vi "Write Handle Drag Starting Msg.vi"(6 "Handle Drag Starting Msg":refnum<class "Handle Drag Starting Msg.lvclass">, 11 "File Explorer Event Filter in":refnum<class "File Explorer Event Filter.lvclass">) -> (3 "File Explorer Event Filter out":refnum<class "File Explorer Event Filter.lvclass">)   [LabVIEW 2020, in "File Explorer.lvlib" / "File Explorer Event Filter.lvclass"]
uses:
  <vilib>/gpm_packages/@cs/file-explorer-extension/Source/File Explorer/File Explorer Event Filter/File Explorer Event Filter.lvclass
  <vilib>/gpm_packages/@cs/file-explorer-extension/Source/File Explorer/File Explorer Messages/Handle Drag Starting Msg/Handle Drag Starting Msg.lvclass
  <vilib>/gpm_packages/@cs/file-explorer-extension/Source/File Explorer/File Explorer Event Filter/File Explorer Event Filter.lvclass/File Explorer Event Filter.ctl
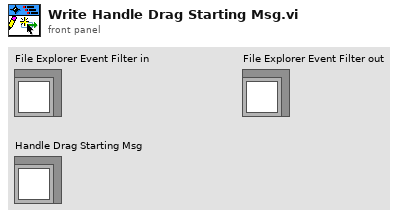
[diagram p1: front panel]
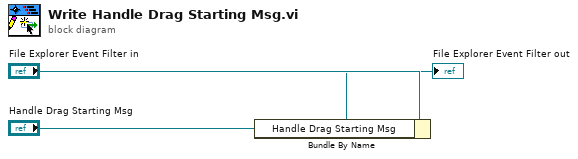
[diagram p0: block diagram]
diagram:
  n1 = Bundle By Name(cluster="File Explorer Event Filter in", "Handle Drag Starting Msg"="Handle Drag Starting Msg") -> (→"File Explorer Event Filter out":refnum<class "File Explorer Event Filter.lvclass">)
